vi "3.2.1.-SubVI RGB a HSV.vi"(9 "B":u8, 10 "G":u8, 11 "R":u8) -> (1 "S":dbl, 2 "V":dbl, 4 "H":dbl)   [LabVIEW 2020]
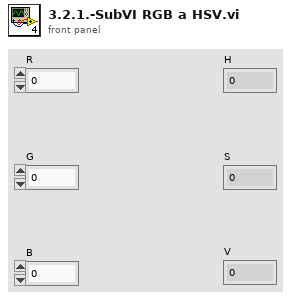
[diagram p1: front panel]
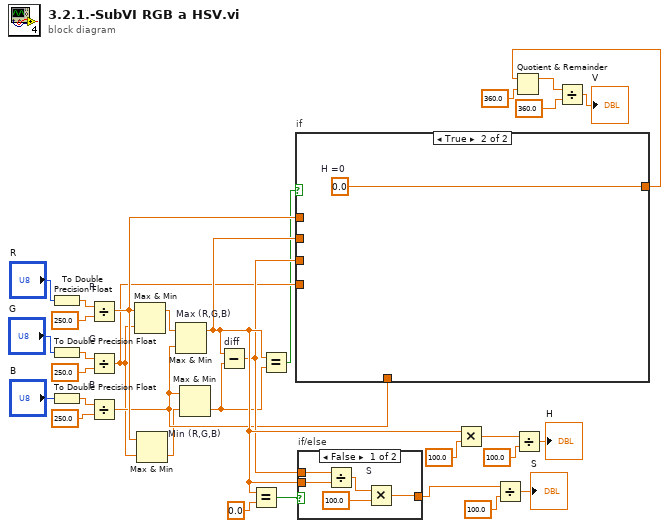
[diagram p0: block diagram]
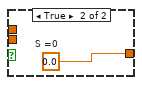
[diagram p2: hidden frame]
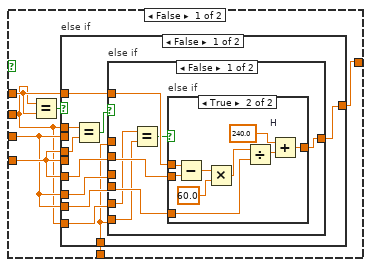
[diagram p3: hidden frame]
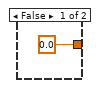
[diagram p4: hidden frame]
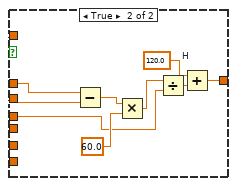
[diagram p5: hidden frame]
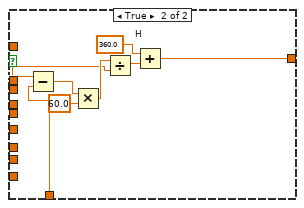
[diagram p6: hidden frame]
diagram:
  n1 = To Double Precision Float(number="R") -> (double precision float=w9:dbl)
  n2 = To Double Precision Float(number="G") -> (double precision float=w10:dbl)
  n3 = To Double Precision Float(number="B") -> (double precision float=w13:dbl)
  n4 = Divide "R"(x=w9, y=250.0) -> (x/y=w29:dbl)
  n5 = Divide "G"(x=w10, y=250.0) -> (x/y=w26:dbl)
  n6 = Divide "B"(x=w13, y=250.0) -> (x/y=w27:dbl)
  n7 = Max & Min(x=w29, y=w26) -> (max(x,y)=w18:dbl)  [unwired: 1 out]
  n8 = Max & Min(x=w29, y=w26) -> (min(x,y)=w19:dbl)  [unwired: 1 out]
  n9 = Max & Min "Max (R,G,B)"(x=w18, y=w27) -> (max(x,y)=w32:dbl)  [unwired: 1 out]
  n10 = Max & Min "Min (R,G,B)"(x=w27, y=w19) -> (min(x,y)=w23:dbl)  [unwired: 1 out]
  n11 = Subtract "diff"(x=w32, y=w23) -> (x-y=w28:dbl)
  n12 = Equal?(x=w32, y=0.0) -> (x = y?=w24:bool)
  n13 = Equal?(x=w32, y=w23) -> (x = y?=w22:bool)
  n14 = case "if" shown="True" w22 {
    tunnel: [w34 w85] -> w30
    tunnel: w26 -> [w36 _]
    tunnel: w27 -> [w39 _]
    tunnel: w28 -> [w35 _]
    tunnel: w32 -> [w33 _]
    tunnel: w29 -> [w37 _]
    frame False {
      n15 = Equal?(x=w33, y=w37) -> (x = y?=w38:bool)
      n16 = case "else if" shown="False" w38 {
        tunnel: w36 -> [_ w78]
        tunnel: w39 -> [w40 w83]
        tunnel: w35 -> [_ w77]
        tunnel: w33 -> [w48 _]
        tunnel: w36 -> [w47 _]
        tunnel: w37 -> [w46 _]
        tunnel: w35 -> [w45 _]
        tunnel: w36 -> [w44 _]
        tunnel: w35 -> [w43 _]
        tunnel: [w42 w76] -> w34
        tunnel: w33 -> [w41 _]
        frame False {
          n17 = Equal?(x=w48, y=w47) -> (x = y?=w49:bool)
          n18 = case "else if" shown="False" w49 {
            tunnel: w40 -> [_ w70]
            tunnel: w46 -> [w56 w69]
            tunnel: w45 -> [_ w68]
            tunnel: w44 -> [w55 _]
            tunnel: w43 -> [w54 _]
            tunnel: [w53 w67] -> w42
            tunnel: w41 -> [w51 _]
            tunnel: w40 -> [w50 _]
            frame False {
              n19 = Equal?(x=w51, y=w50) -> (x = y?=w52:bool)
              n20 = case "else if" shown="True" w52 {
                tunnel: w56 -> [_ w61]
                tunnel: w55 -> [_ w60]
                tunnel: w54 -> [_ w59]
                tunnel: [0.0 w58] -> w53
                frame False {
                }
                frame True {
                  n21 = Subtract(x=w61, y=w60) -> (x-y=w64:dbl)
                  n22 = Multiply(x=w64, y=60.0) -> (x*y=w65:dbl)
                  n23 = Divide(x=w65, y=w59) -> (x/y=w66:dbl)
                  n24 = Add "H"(x=240.0, y=w66) -> (x+y=w58:dbl)
                }
              }
            }
            frame True {
              n25 = Subtract(x=w70, y=w69) -> (x-y=w74:dbl)
              n26 = Multiply(x=w74, y=60.0) -> (x*y=w73:dbl)
              n27 = Divide(x=w73, y=w68) -> (x/y=w72:dbl)
              n28 = Add "H"(x=120.0, y=w72) -> (x+y=w67:dbl)
            }
          }
        }
        frame True {
          n29 = Subtract(x=w78, y=w83) -> (x-y=w82:dbl)
          n30 = Multiply(x=w82, y=60.0) -> (x*y=w81:dbl)
          n31 = Divide(x=w81, y=w77) -> (x/y=w80:dbl)
          n32 = Add "H"(x=360.0, y=w80) -> (x+y=w76:dbl)
        }
      }
    }
    frame True {
      w85 = 0.0  # H =0
    }
  }
  n33 = case "if/else" shown="False" w24 {
    tunnel: [w86 w91] -> w31
    tunnel: w28 -> [w90 _]
    tunnel: w32 -> [w89 _]
    frame False {
      n34 = Divide(x=w90, y=w89) -> (x/y=w87:dbl)
      n35 = Multiply "S"(x=w87, y=100.0) -> (x*y=w86:dbl)
    }
    frame True {
      w91 = 0.0  # S =0
    }
  }
  n36 = Multiply(x=w32, y=100.0) -> (x*y=w21:dbl)
  n37 = Divide(x=w31, y=100.0) -> (x/y=→"S":dbl)
  n38 = Quotient & Remainder(x=w30, y=360.0) -> (x-y*floor(x/y)=w3:dbl)  [unwired: 1 out]
  n39 = Divide(x=w21, y=100.0) -> (x/y=→"H":dbl)
  n40 = Divide(x=w3, y=360.0) -> (x/y=→"V":dbl)
